vi "CreatePrivateEvents.vi"(8 "error in (no error)":errorcluster, 11 "DAQ_Manager":refnum<class "DAQ_Manager.lvclass">) -> (0 "error out":errorcluster, 3 "DAQ_Manager out":refnum<class "DAQ_Manager.lvclass">)   [LabVIEW 2016, in "DAQ_Manager.lvclass"]
doc: "---------------------------------------------------------------\nJKI State Machine Objects™\nhttp://jki.net/state-machine-objects/\nCopyright (C) 2005-2015, JKI <info@jki.net>\nALL RIGHTS RESERVEDJKI State Machine Objects (SMO) 1.0.0.4\nJKI - JKI\nCopyright (c) 2015, JKI"
uses:
  DAQ_Manager.lvclass
  Typedefs/PrivateEvents--DAQ_Manager.setWaveform.ctl
  Typedefs/PrivateEvents--DAQ_Manager.DAQ_Manager.setDAQConfig.ctl
  DAQ_Manager.lvclass/DAQ_Manager.ctl
  <vilib>/JKI/JKI SMO/SMO/SMO.lvclass
panel:
  # "For instructions on how to use the JKI State Machine Objects, examples and video tutorials, visit:\nhttp://jki.net/state-machine-objects/\n\nJKI State Machine Objects™\nhttp://jki.net/state-machine-objects/\nCopyright (C) 2005-2015, JKI <info@jki.net>\nALL RIGHTS RESERVED"
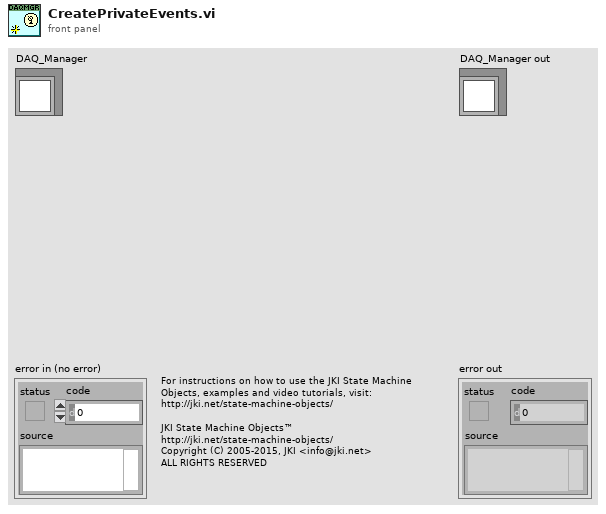
[diagram p1: front panel]
types:
  T1 = typedef "DAQ_Manager.lvclass/PrivateEvents--DAQ_Manager.DAQ_Manager.setDAQConfig.ctl" = cluster{"DAQ.Config (AI)":cluster{"Channels":string, "DAQ_Type":enum16{"AI", "AO"}, "minimum value":dbl, "maximum value":dbl, "DAQ_SamplingInfo":cluster{"Fs":dbl, "#s":i32}, "DAQ_SamplingMode":enum16{"Continuous", "Finite"}}[], "DAQmx.AI.config":cluster{"AI.Coupling":i32, "input terminal configuration ":i32}[], "DAQ.Config (AO)":cluster{"Channels":string, "DAQ_Type":enum16{"AI", "AO"}, "minimum value":dbl, "maximum value":dbl, "DAQ_SamplingInfo":cluster{"Fs":dbl, "#s":i32}, "DAQ_SamplingMode":enum16{"Continuous", "Finite"}}[], "DAQmx.AO.config":cluster{"output terminal configuration":i32}[]}
  T2 = typedef "DAQ_Manager.lvclass/PrivateEvents--DAQ_Manager.setWaveform.ctl" = waveform(dbl)[]
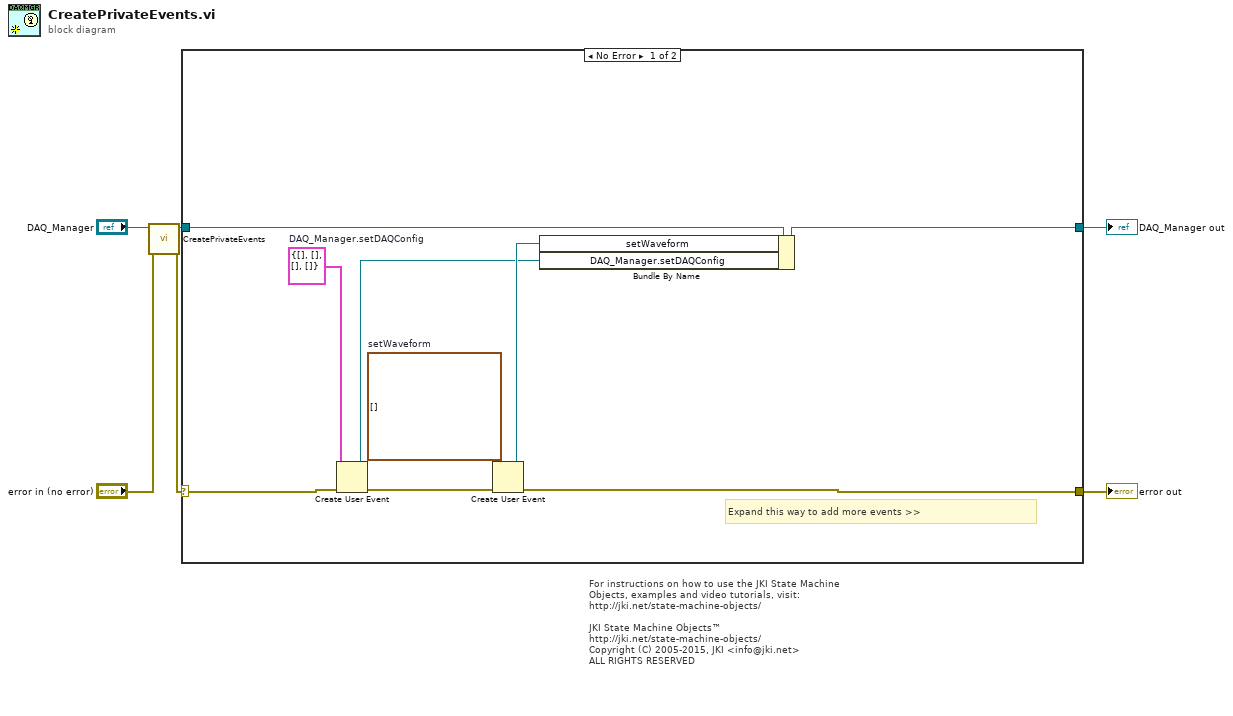
[diagram p0: block diagram]
diagram:
  # "For instructions on how to use the JKI State Machine Objects, examples and video tutorials, visit:\nhttp://jki.net/state-machine-objects/\n\nJKI State Machine Objects™\nhttp://jki.net/state-machine-objects/\nCopyright (C) 2005-2015, JKI <info@jki.net>\nALL RIGHTS RESERVED"
  n1 = call-parent "CreatePrivateEvents.vi"("error in (no error)"="error in (no error)", "SMO"="DAQ_Manager") -> ("error out"=w1:errorcluster, "SMO out"=w3:refnum<class "DAQ_Manager.lvclass">)  [unwired: 8 in]
  n2 = case shown="No Error" w1 {
    selector: w1 -> [w14 w17]
    tunnel: [w12 w17] -> w5
    tunnel: [w13 w16] -> w6
    tunnel: w3 -> [w15 w16]
    frame No Error {
      w8 = T1 {"DAQ.Config (AI)"=[], "DAQmx.AI.config"=[], "DAQ.Config (AO)"=[], "DAQmx.AO.config"=[]}  # DAQ_Manager.setDAQConfig
      w11 = T2 []  # setWaveform
      # "Expand this way to add more events >>"
      n3 = Create User Event(user event datatype=w8, error in=w14) -> (user event=w7:refnum<user-event>, error out=w9:errorcluster)
      n4 = Create User Event(user event datatype=w11, error in=w9) -> (user event=w10:refnum<user-event>, error out=w12:errorcluster)
      n5 = Bundle By Name(cluster=w15, "setWaveform"=w10, "DAQ_Manager.setDAQConfig"=w7) -> (w13:refnum<class "DAQ_Manager.lvclass">)
    }
    frame Error {
    }
  }
  "error out" <- w5
  "DAQ_Manager out" <- w6
